vi "DeltaFour.vi"() -> ()   [LabVIEW 2012]
uses:
  <vilib>/NXT/Subs/MotorOutput.ctl
  <vilib>/NXT/NXT Controls/ConnectionType.ctl
  <vilib>/NXT/Block Support/NXT_InputPort.ctl
panel:
  in  "?":bool
  out "?":bool
  out "?":bool
  out "?":bool
  out "?":bool
  out "?":bool
  out "?":bool
  out "?":bool
  out "?":bool
  out "?":bool
  out "?":bool
  out "?":bool
  out "?":bool
  out "?":bool
  out "?":bool
  out "?":bool
  out "?":bool
  out "?":bool
  out "?":bool
  out "?":bool
  out "2D-Image":picture
  out "3D-Image":picture
  out "?":bool
  out "?":bool
  out "?":bool
  out "?":bool
  out "?":bool
  out "Progress":u8(slide) scale=0.0..100.0
  out "Motor B2":dbl
  out "Motor B1":dbl
  out "Motor A2":dbl
  out "Motor A1":dbl
  out "?":bool
  out "?":bool
  out "?":bool
  in  "Input molecule name or extended sum formula:":string
  out "Status:":string
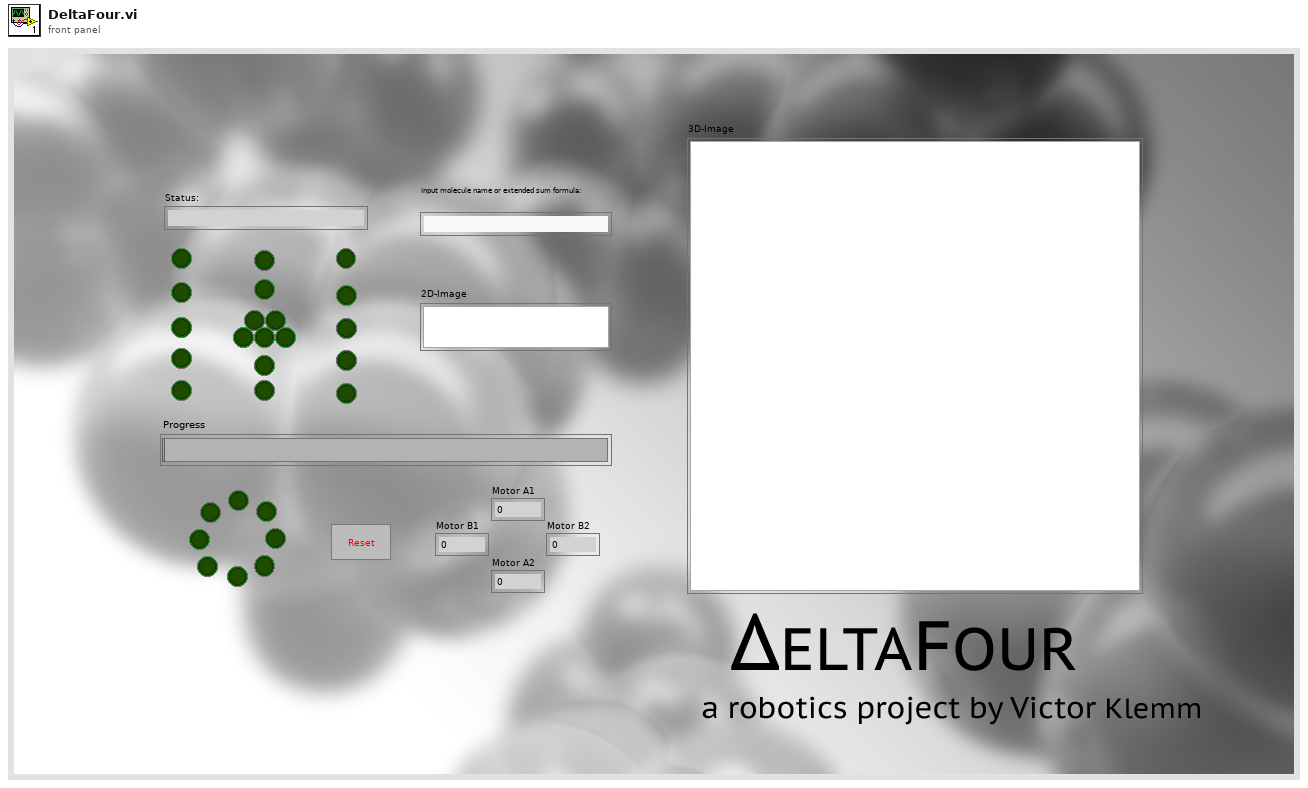
[diagram p1: front panel]
types:
  T1 = typedef "ConnectionType.ctl" = enum16{"Bluetooth", "USB", "WiFi"}
  T2 = typedef "LVHSConnector.ctl" = refnum<class "BrickReference.lvclass">
  T3 = typedef "imagedata.ctl" = cluster{"image type":i32, "image depth":i32, "image":u8[], "mask":u8[], "colors":u32[], "Rectangle":cluster{"left":i16, "top":i16, "right":i16, "bottom":i16}}
  T4 = typedef "MotorOutput.ctl" = u8
  T5 = typedef "NXT_InputPort.ctl" = u8
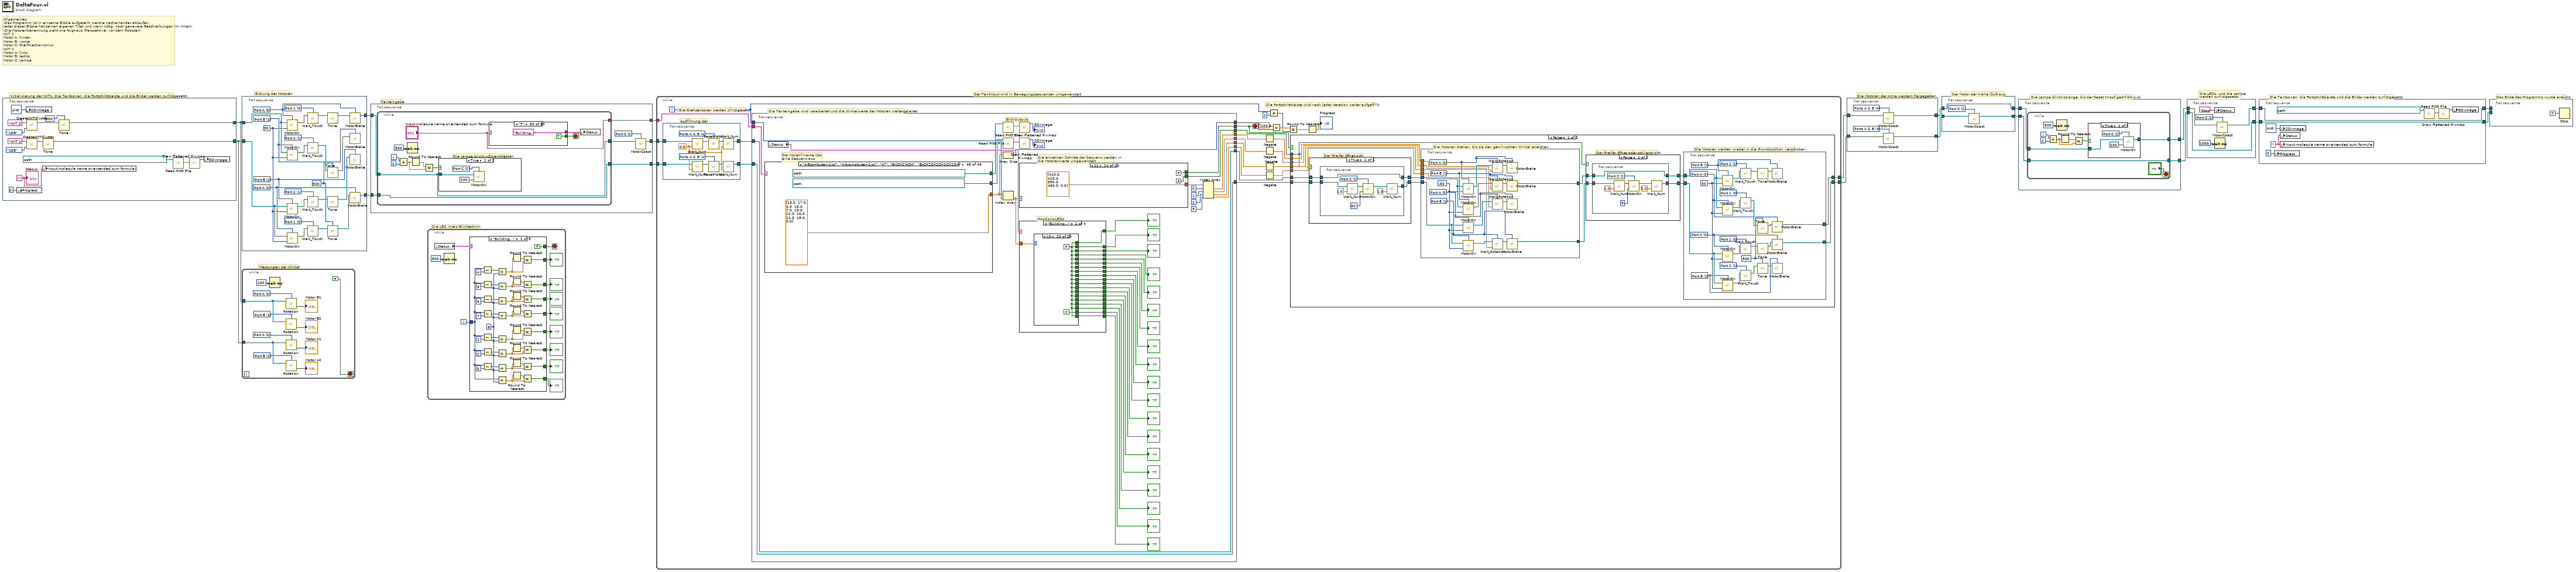
[diagram p0: block diagram]
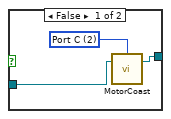
[diagram p2: hidden frame]
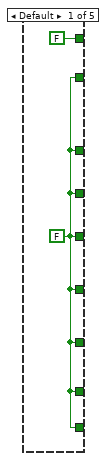
[diagram p3: hidden frame]
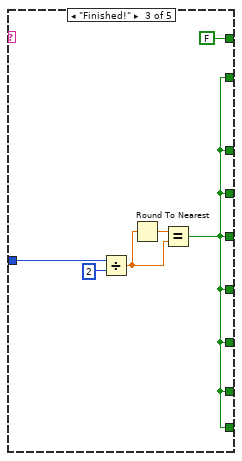
[diagram p4: hidden frame]
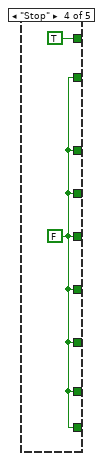
[diagram p5: hidden frame]
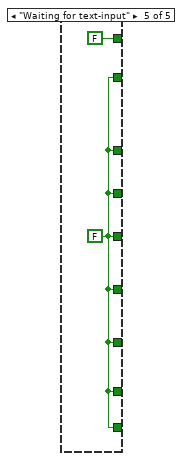
[diagram p6: hidden frame]
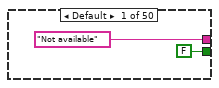
[diagram p7: hidden frame]
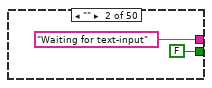
[diagram p8: hidden frame]
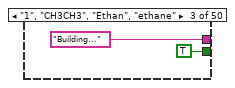
[diagram p9: hidden frame]
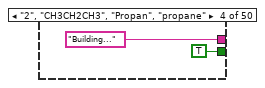
[diagram p10: hidden frame]
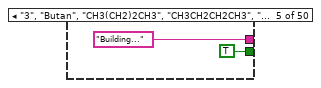
[diagram p11: hidden frame]
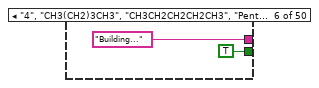
[diagram p12: hidden frame]
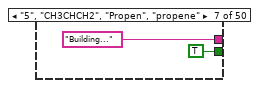
[diagram p13: hidden frame]
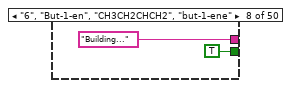
[diagram p14: hidden frame]
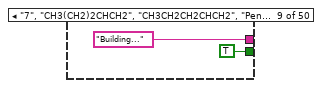
[diagram p15: hidden frame]
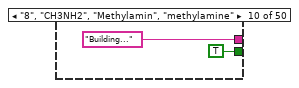
[diagram p16: hidden frame]
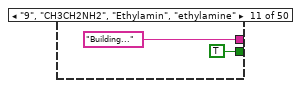
[diagram p17: hidden frame]
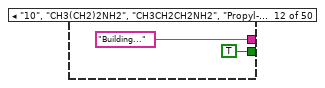
[diagram p18: hidden frame]
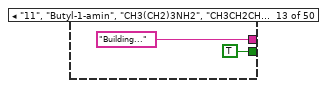
[diagram p19: hidden frame]
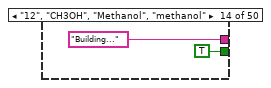
[diagram p20: hidden frame]
diagram:
  # "Eichung der Motoren"
  # "Der Textinput wird in Bewegungssequenzen umgewandelt"
  # "Die Textboxen, die Fortschrittsleiste und die Bilder werden zurŸckgesetzt."
  # "Das Ende des Programms wurde erreicht."
  # "Allgemeines:\n-Das Programm ist in einzelne Blšcke aufgeteilt, welche nacheinander ablaufen.\nJeder dieser Blšcke hat seinen eigenen Titel und wenn nštig, noch genauere Beschreibungen im Innern,\n-Die Motorenbenennung sieht wie folgt aus (Perspektive: vor dem Roboter):\nNXT 1\nMotor A: hinten\nMotor B: vorne\nMotor C: Greifmechanismus\nNXT 2\nMotor A: links\nMotor B: rechts\nMotor C: Lampe"
  # "Die Motoren der Arme werdem freigegeben."
  # "Die Lampe blinkt solange, bis der Reset Knopf gedrŸckt wird."
  # "Der Motor der Kralle lŠuft aus."
  # "Messungen der Winkel"
  # "Die LEDs, und die Lampe\nwerden zurŸckgesetzt"
  # "Texteingabe"
  # "Initialisierung der NXTs. Die Textboxen, die Fortschrittsleiste und die Bilder werden zurŸckgesetzt."
  # "Die LED -Kreis Blinktechnik"
  n1 = flat-sequence {
    tunnel: [w31] -> w10
    tunnel: [w29] -> w11
    frame #0 {
      w28 = "" ("Status:")
      n2 = local write "Progress"(u8 0 ("Progress")) -> ()
      n3 = local write "2D-Image"(picture data[5B] ("2D")) -> ()
      n4 = call <vilib>:"CreateNXTCluster.vi"("Connection Type"=ConnectionType."USB", "NXT name"="NXT 2") -> ("NXT"=w30:T2)  [unwired: 2 in]
      n5 = call <vilib>:"CreateNXTCluster.vi"("Connection Type"=ConnectionType."USB", "NXT name"="NXT 1") -> ("NXT"=w32:T2)  [unwired: 2 in]
      n6 = local write "Input molecule name or extended sum formula:"(w28) -> ()
      n7 = call <vilib>:"Tone.vi"("NXT"=w32) -> ("NXT"=w31:T2)  [unwired: 3 in]
      n8 = call <vilib>:"Tone.vi"("NXT"=w30, "Tone (440 Hz)"=u16 500) -> ("NXT"=w29:T2)  [unwired: 2 in]
      n9 = call <vilib>:"Read PNG File.vi"("path to PNG file"=path "/Macintosh HD/Users/victor_klemm/Documents/ÆFour Molecules/3D Molecules/0.png") -> ("image data"=w22:T3)  [unwired: 8 in, 2 out]
      n10 = call <vilib>:"Draw Flattened Pixmap.vi"("image data"=w22) -> ("new picture"=w20:picture)  [unwired: 8 in]
      n11 = local write "3D-Image"(w20) -> ()
      "Status:" <- w28
    }
  }
  n12 = flat-sequence {
    tunnel: w11 -> [w56]
    tunnel: w10 -> [w55]
    tunnel: [w42] -> w13
    tunnel: [w41] -> w12
    frame #0 {
      w35 = u16 500 ("Tone (440 Hz)")
      w38 = T4 1 items=["Port A"=0, "Port B"=1, "Port C"=2, "Ports A & B"=4, "Ports A & C"=5, "Ports B & C"=6, "All Ports"=3] ("Output Port (All Ports)")
      w51 = T5 1 items=["Port 1", "Port 2", "Port 3", "Port 4"] ("Port (Port 1)")
      w50 = T5 0 items=["Port 1", "Port 2", "Port 3", "Port 4"] ("Port (Port 1)")
      w36 = T4 1 items=["Port A"=0, "Port B"=1, "Port C"=2, "Ports A & B"=4, "Ports A & C"=5, "Ports B & C"=6, "All Ports"=3] ("Output Port (All Ports)")
      w37 = T4 0 items=["Port A"=0, "Port B"=1, "Port C"=2, "Ports A & B"=4, "Ports A & C"=5, "Ports B & C"=6, "All Ports"=3] ("Output Port (All Ports)")
      w39 = T5 1 items=["Port 1", "Port 2", "Port 3", "Port 4"] ("Port (Port 1)")
      w52 = T5 0 items=["Port 1", "Port 2", "Port 3", "Port 4"] ("Port (Port 1)")
      w43 = 30 ("Power (75)")
      w40 = T4 0 items=["Port A"=0, "Port B"=1, "Port C"=2, "Ports A & B"=4, "Ports A & C"=5, "Ports B & C"=6, "All Ports"=3] ("Output Port (All Ports)")
      n13 = call <vilib>:"MotorOn.vi"("Power (75)"=w43, "NXT"=w56, "Output Port (All Ports)"=w40) -> ("NXT"=w60:T2)  [unwired: 1 in]
      n14 = call <vilib>:"MotorOn.vi"("Power (75)"=w43, "NXT"=w56, "Output Port (All Ports)"=w38) -> ("NXT"=w59:T2)  [unwired: 1 in]
      n15 = call <vilib>:"MotorOn.vi"("Power (75)"=w43, "NXT"=w55, "Output Port (All Ports)"=w36) -> ("NXT"=w57:T2)  [unwired: 1 in]
      n16 = call <vilib>:"MotorOn.vi"("Power (75)"=w43, "NXT"=w55, "Output Port (All Ports)"=w37) -> ("NXT"=w58:T2)  [unwired: 1 in]
      n17 = call <vilib>:"Wait_Touch.vi"("NXT"=w60, "Port (Port 1)"=w52) -> ("NXT"=w54:T2)  [unwired: 2 in]
      n18 = call <vilib>:"Wait_Touch.vi"("NXT"=w59, "Port (Port 1)"=w39) -> ("NXT"=w49:T2)  [unwired: 2 in]
      n19 = call <vilib>:"Wait_Touch.vi"("NXT"=w57, "Port (Port 1)"=w51) -> ("NXT"=w47:T2)  [unwired: 2 in]
      n20 = call <vilib>:"Wait_Touch.vi"("NXT"=w58, "Port (Port 1)"=w50) -> ("NXT"=w45:T2)  [unwired: 2 in]
      n21 = call <vilib>:"Tone.vi"("NXT"=w54) -> ("NXT"=w53:T2)  [unwired: 3 in]
      n22 = call <vilib>:"Tone.vi"("NXT"=w49, "Tone (440 Hz)"=w35) -> ("NXT"=w48:T2)  [unwired: 2 in]
      n23 = call <vilib>:"Tone.vi"("NXT"=w47) -> ("NXT"=w46:T2)  [unwired: 3 in]
      n24 = call <vilib>:"Tone.vi"("NXT"=w45, "Tone (440 Hz)"=w35) -> ("NXT"=w44:T2)  [unwired: 2 in]
      n25 = call <vilib>:"MotorBrake.vi"("NXT"=w53, "Port (All Ports)"=w40) -> ("NXT"=w42:T2)  [unwired: 2 in]
      n26 = call <vilib>:"MotorBrake.vi"("NXT"=w48, "Port (All Ports)"=w38) -> ()  [unwired: 2 in, 1 out]
      n27 = call <vilib>:"MotorBrake.vi"("NXT"=w46, "Port (All Ports)"=w36) -> ()  [unwired: 2 in, 1 out]
      n28 = call <vilib>:"MotorBrake.vi"("NXT"=w44, "Port (All Ports)"=w37) -> ("NXT"=w41:T2)  [unwired: 2 in]
    }
  }
  n29 = while {
    tunnel: w11 -> [w68]
    tunnel: w10 -> [w67]
    stop <- FALSE stop-if-true
    w70 = T4 1 items=["Port A"=0, "Port B"=1, "Port C"=2, "Ports A & B"=4, "Ports A & C"=5, "Ports B & C"=6, "All Ports"=3] ("Output Port (All Ports)")
    w69 = T4 0 items=["Port A"=0, "Port B"=1, "Port C"=2, "Ports A & B"=4, "Ports A & C"=5, "Ports B & C"=6, "All Ports"=3] ("Output Port (All Ports)")
    w72 = T4 1 items=["Port A"=0, "Port B"=1, "Port C"=2, "Ports A & B"=4, "Ports A & C"=5, "Ports B & C"=6, "All Ports"=3] ("Output Port (All Ports)")
    w71 = T4 0 items=["Port A"=0, "Port B"=1, "Port C"=2, "Ports A & B"=4, "Ports A & C"=5, "Ports B & C"=6, "All Ports"=3] ("Output Port (All Ports)")
    n30 = Wait (ms)(milliseconds to wait=u32 100) -> ()  [unwired: 1 out]
    n31 = call <vilib>:"Rotation.vi"("NXT"=w68, "Port (Port A)"=w71) -> ("Angle of Rotation"=→"Motor B1":i32)  [unwired: 1 in, 1 out]
    n32 = call <vilib>:"Rotation.vi"("NXT"=w68, "Port (Port A)"=w72) -> ("Angle of Rotation"=→"Motor B2":i32)  [unwired: 1 in, 1 out]
    n33 = call <vilib>:"Rotation.vi"("NXT"=w67, "Port (Port A)"=w69) -> ("Angle of Rotation"=→"Motor A1":i32)  [unwired: 1 in, 1 out]
    n34 = call <vilib>:"Rotation.vi"("NXT"=w67, "Port (Port A)"=w70) -> ("Angle of Rotation"=→"Motor A2":i32)  [unwired: 1 in, 1 out]
  }
  n35 = flat-sequence {
    tunnel: w12 -> [w77]
    tunnel: [w79] -> w19
    tunnel: [w78] -> w8
    tunnel: [w74] -> w7
    tunnel: w13 -> [w76]
    frame #0 {
      w73 = T4 2 items=["Port A"=0, "Port B"=1, "Port C"=2, "Ports A & B"=4, "Ports A & C"=5, "Ports B & C"=6, "All Ports"=3] ("Port (All Ports)")
      n36 = while {
        tunnel: ["Input molecule name or extended sum formula:"] -> w79
        tunnel: [w89] -> w78
        tunnel: w77 -> [w89]
        tunnel: w76 -> [w84]
        tunnel: [w84] -> w75
        i -> [w83]
        stop <- w82 stop-if-true
        # "Die Lampe blinkt wŠhrenddessen"
        n37 = Divide(x=w83, y=2) -> (x/y=w86:dbl)
        n38 = Wait (ms)(milliseconds to wait=u32 500) -> ()  [unwired: 1 out]
        n39 = Round To Nearest(number=w86) -> (nearest integer value=w87:dbl)
        n40 = Equal?(x=w87, y=w86) -> (x = y?=w85:bool)
        n41 = case shown="True" w85 {
          tunnel: w84 -> [w191 w194]
          frame False {
            w192 = T4 2 items=["Port A"=0, "Port B"=1, "Port C"=2, "Ports A & B"=4, "Ports A & C"=5, "Ports B & C"=6, "All Ports"=3] ("Port (All Ports)")
            n42 = call <vilib>:"MotorCoast.vi"("NXT"=w191, "Port (All Ports)"=w192) -> ()  [unwired: 2 in, 1 out]
          }
          frame True {
            w193 = T4 2 items=["Port A"=0, "Port B"=1, "Port C"=2, "Ports A & B"=4, "Ports A & C"=5, "Ports B & C"=6, "All Ports"=3] ("Output Port (All Ports)")
            n43 = call <vilib>:"MotorOn.vi"("Power (75)"=100, "NXT"=w194, "Output Port (All Ports)"=w193) -> ()  [unwired: 1 in, 1 out]
          }
        }
        n44 = case shown="\"T\"" "Input molecule name or extended sum formula:" {
          tunnel: ["Not available" ("Status") "Waiting for text-input" ("Status") "Building..." ("Status") "Building..." ("Status") "Building..." ("Status") "Building..." ("Status") "Building..." ("Status") "Building..." ("Status") "Building..." ("Status") "Building..." ("Status") "Building..." ("Status") "Building..." ("Status") "Building..." ("Status") "Building..." ("Status") "Building..." ("Status") "Building..." ("Status") "Building..." ("Status") "Building..." ("Status") "Building..." ("Status") "Building..." ("Status") "Building..." ("Status") "Building..." ("Status") "Building..." ("Status") "Building..." ("Status") "Building..." ("Status") "Building..." ("Status") "Building..." ("Status") "Building..." ("Status") "Building..." ("Status") "Building..." ("Status") "Building..." ("Status") "Building..." ("Status") "Building..." ("Status") "Building..." ("Status") "Building..." ("Status") "Building..." ("Status") "Building..." ("Status") "Building..." ("Status") "Building..." ("Status") "Building..." ("Status") "Building..." ("Status") "Building..." ("Status") "Building..." ("Status") "Building..." ("Status") "Building..." ("Status") "Building..." ("Status") "Building..." ("Status") "Building..." ("Status") "Building..." ("Status") "Building..." ("Status")] -> w80
          tunnel: [FALSE FALSE TRUE TRUE TRUE TRUE TRUE TRUE TRUE TRUE TRUE TRUE TRUE TRUE TRUE TRUE TRUE TRUE TRUE TRUE TRUE TRUE TRUE TRUE TRUE TRUE TRUE TRUE TRUE TRUE TRUE TRUE TRUE TRUE TRUE TRUE TRUE TRUE TRUE TRUE TRUE TRUE TRUE TRUE TRUE TRUE TRUE TRUE TRUE TRUE] -> w82
          frame Default {
          }
          frame "" {
          }
          frame "1", "CH3CH3", "Ethan", "ethane" {
          }
          frame "2", "CH3CH2CH3", "Propan", "propane" {
          }
          frame "3", "Butan", "CH3(CH2)2CH3", "CH3CH2CH2CH3", "butane" {
          }
          frame "4", "CH3(CH2)3CH3", "CH3CH2CH2CH2CH3", "Pentan", "pentane" {
          }
          frame "5", "CH3CHCH2", "Propen", "propene" {
          }
          frame "6", "But-1-en", "CH3CH2CHCH2", "but-1-ene" {
          }
          frame "7", "CH3(CH2)2CHCH2", "CH3CH2CH2CHCH2", "Pent-1-en", "pent-1-ene" {
          }
          frame "8", "CH3NH2", "Methylamin", "methylamine" {
          }
          frame "9", "CH3CH2NH2", "Ethylamin", "ethylamine" {
          }
          frame "10", "CH3(CH2)2NH2", "CH3CH2CH2NH2", "Propyl-1-amin", "propyl-1-amine" {
          }
          frame "11", "Butyl-1-amin", "CH3(CH2)3NH2", "CH3CH2CH2CH2NH2", "butyl-1-amine" {
          }
          frame "12", "CH3OH", "Methanol", "methanol" {
          }
          frame "13", "CH3CH2OH", "Ethanol", "ethanol" {
          }
          frame "14", "CH3(CH2)2OH", "CH3CH2CH2OH", "Propanol", "propanol" {
          }
          frame "15", "Butanol", "CH3(CH2)3OH", "CH3CH2CH2CH2OH", "butanol" {
          }
          frame "16", "CH3CH2Cl", "Chlorethan", "chloroethane" {
          }
          frame "1-Chlorpropan", "1-chloropropane", "17", "CH3(CH2)2Cl", "CH3CH2CH2Cl" {
          }
          frame "1-Chlorbutan", "1-chlorobutane", "18", "CH3(CH2)3Cl", "CH3CH2CH2CH2Cl" {
          }
          frame "1-Chlorpentan", "1-chloropentane", "19", "CH3(CH2)4Cl", "CH3CH2CH2CH2CH2Cl" {
          }
          frame "20", "CH3CH2I", "Iodethan", "iodoethane" {
          }
          frame "1-Iodpropan", "1-iodopropane", "21", "CH3(CH2)2I", "CH3CH2CH2I" {
          }
          frame "1-Iodbutan", "1-iodobutane", "22", "CH3(CH2)3I", "CH3CH2CH2CH2I" {
          }
          frame "1-Iodpentan", "1-iodopentane", "23", "CH3(CH2)4I", "CH3CH2CH2CH2CH2I" {
          }
          frame "24", "Bromethan", "CH3CH2Br", "bromoethane" {
          }
          frame "1-Brompropan", "1-bromopropane", "25", "CH3(CH2)2Br", "CH3CH2CH2Br" {
          }
          frame "1-Brombutan", "1-bromobutane", "26", "CH3(CH2)3Br", "CH3CH2CH2CH2Br" {
          }
          frame "1-Brompentan", "1-bromopentane", "27", "CH3(CH2)4Br", "CH3CH2CH2CH2CH2Br" {
          }
          frame "28", "CH2CHNH2", "Ethenylamin", "ethenylamine" {
          }
          frame "29", "But-3-enyl-1-amin", "CH2CH(CH2)2NH2", "CH2CHCH2CH2NH2", "but-3-enyl-1-amine" {
          }
          frame "30", "CH2CHOH", "Ethenol", "ethenol" {
          }
          frame "31", "But-3-en-1-ol", "CH2CH(CH2)2OH", "CH2CHCH2CH2OH", "but-3-en-1-ol" {
          }
          frame "3-Chlorprop-1-en", "3-chloroprop-1-ene", "32", "CH2CHCH2Cl" {
          }
          frame "33", "5-Chlorpent-1-en", "5-chloropent-1-ene", "CH2CH(CH2)3Cl", "CH2CHCH2CH2CH2Cl" {
          }
          frame "3-Iodprop-1-en", "3-iodoprop-1-ene", "34", "CH2CHCH2I" {
          }
          frame "35", "5-Iodpent-1-en", "5-iodopent-1-ene", "CH2CH(CH2)3I", "CH2CHCH2CH2CH2I" {
          }
          frame "3-Bromprop-1-en", "3-bromoprop-1-ene", "36", "CH2CHCH2Br" {
          }
          frame "37", "5-Brompent-1-en", "5-bromopent-1-ene", "CH2CH(CH2)3Br", "CH2CHCH2CH2CH2Br" {
          }
          frame "38", "Aminomethanol", "NH2CH2OH", "aminomethanol" {
          }
          frame "3-Aminopropan-1-ol", "3-aminopropan-1-ol", "39", "NH2(CH2)3OH", "NH2CH2CH2CH2OH" {
          }
          frame "40", "Methandiol", "OHCH2OH", "methanediol" {
          }
          frame "41", "OH(CH2)3OH", "OHCH2CH2CH2OH", "Propan-1,3-diol", "propane-1,3-diol" {
          }
          frame "2-Chlorethan-1-ol", "2-chloroethan-1-ol", "42", "ClCH2CH2OH" {
          }
          frame "4-Chlorbutan-1-ol", "4-chlorobutan-1-ol", "43", "Cl(CH2)4OH", "ClCH2CH2CH2CH2OH" {
          }
          frame "2-Iodethan-1-ol", "2-iodoethan-1-ol", "44", "ICH2CH2OH" {
          }
          frame "4-Iodbutan-1-ol", "4-iodobutan-1-ol", "45", "I(CH2)4OH", "ICH2CH2CH2CH2OH" {
          }
          frame "2-Bromethan-1-ol", "2-bromoethan-1-ol", "46", "BrCH2CH2OH" {
          }
          frame "4-Brombutan-1-ol", "4-bromobutan-1-ol", "47", "Br(CH2)4OH", "BrCH2CH2CH2CH2OH" {
          }
          frame "T" {
          }
        }
        n45 = local write "Status:"(w80) -> ()
      }
      n46 = call <vilib>:"MotorCoast.vi"("NXT"=w75, "Port (All Ports)"=w73) -> ("NXT"=w74:T2)  [unwired: 2 in]
    }
  }
  n47 = while {
    i -> [w207]
    stop <- w205 stop-if-true
    n48 = local read "Status:"() -> (w204:string)
    n49 = Wait (ms)(milliseconds to wait=u32 500) -> ()  [unwired: 1 out]
    n50 = case shown="\"Building...\"" w204 {
      tunnel: w207 -> [_ w211 w253 _ _]
      tunnel: [FALSE FALSE FALSE TRUE FALSE] -> w205
      tunnel: [w208 w239 w251 w257 w259] -> w203
      tunnel: [w208 w238 w251 w257 w259] -> w202
      tunnel: [w208 w237 w251 w257 w259] -> w201
      tunnel: [w208 w232 w251 w257 w259] -> w200
      tunnel: [w208 w228 w251 w257 w259] -> w199
      tunnel: [w208 w222 w251 w257 w259] -> w198
      tunnel: [w208 w217 w251 w257 w259] -> w197
      tunnel: [w208 w212 w251 w257 w259] -> w196
      frame Default {
        w208 = FALSE ("stop? (T)")
      }
      frame "Building..." {
        w210 = 8 ("y")
        n51 = Subtract(x=w211, y=4) -> (x-y=w230:i32)
        n52 = Subtract(x=w211, y=5) -> (x-y=w225:i32)
        n53 = Subtract(x=w211, y=6) -> (x-y=w220:i32)
        n54 = Subtract(x=w211, y=7) -> (x-y=w215:i32)
        n55 = Subtract(x=w211, y=1) -> (x-y=w246:i32)
        n56 = Subtract(x=w211, y=2) -> (x-y=w242:i32)
        n57 = Subtract(x=w211, y=3) -> (x-y=w234:i32)
        n58 = Divide(x=w230, y=w210) -> (x/y=w231:dbl)
        n59 = Divide(x=w225, y=w210) -> (x/y=w226:dbl)
        n60 = Divide(x=w220, y=w210) -> (x/y=w221:dbl)
        n61 = Divide(x=w215, y=w210) -> (x/y=w216:dbl)
        n62 = Divide(x=w246, y=w210) -> (x/y=w247:dbl)
        n63 = Divide(x=w242, y=w210) -> (x/y=w243:dbl)
        n64 = Divide(x=w234, y=w210) -> (x/y=w235:dbl)
        n65 = Divide(x=w211, y=w210) -> (x/y=w249:dbl)
        n66 = Round To Nearest(number=w231) -> (nearest integer value=w227:dbl)
        n67 = Round To Nearest(number=w226) -> (nearest integer value=w223:dbl)
        n68 = Round To Nearest(number=w221) -> (nearest integer value=w218:dbl)
        n69 = Round To Nearest(number=w216) -> (nearest integer value=w213:dbl)
        n70 = Round To Nearest(number=w247) -> (nearest integer value=w248:dbl)
        n71 = Round To Nearest(number=w243) -> (nearest integer value=w244:dbl)
        n72 = Round To Nearest(number=w235) -> (nearest integer value=w236:dbl)
        n73 = Round To Nearest(number=w249) -> (nearest integer value=w250:dbl)
        n74 = Equal?(x=w227, y=w231) -> (x = y?=w228:bool)
        n75 = Equal?(x=w223, y=w226) -> (x = y?=w222:bool)
        n76 = Equal?(x=w218, y=w221) -> (x = y?=w217:bool)
        n77 = Equal?(x=w213, y=w216) -> (x = y?=w212:bool)
        n78 = Equal?(x=w248, y=w247) -> (x = y?=w237:bool)
        n79 = Equal?(x=w244, y=w243) -> (x = y?=w238:bool)
        n80 = Equal?(x=w236, y=w235) -> (x = y?=w232:bool)
        n81 = Equal?(x=w250, y=w249) -> (x = y?=w239:bool)
      }
      frame "Finished!" {
        n82 = Divide(x=w253, y=2) -> (x/y=w255:dbl)
        n83 = Round To Nearest(number=w255) -> (nearest integer value=w252:dbl)
        n84 = Equal?(x=w252, y=w255) -> (x = y?=w251:bool)
      }
      frame "Stop" {
        w257 = FALSE ("stop? (T)")
      }
      frame "Waiting for text-input" {
        w259 = FALSE ("stop? (T)")
      }
    }
    "?" <- w203
    "?" <- w202
    "?" <- w201
    "?" <- w197
    "?" <- w196
    "?" <- w200
    "?" <- w199
    "?" <- w198
  }
  n85 = while {
    tunnel: w8 -> [w285]
    tunnel: w7 -> [w284]
    tunnel: w19 -> [w281]
    tunnel: [w262] -> w4
    tunnel: [w261] -> w5
    i -> [w273]
    stop <- w279 stop-if-true
    # "Die Fortschrittsleiste wird nach jeder Iteration weiter aufgefŸllt."
    # "AusfŸhrung der"
    # "Die Texteingabe wird verarbeitet und die Winkelwerte der Motoren weitergeleitet"
    # "Die Drehsensoren werden zŸrickgesetzt"
    n86 = flat-sequence {
      tunnel: w285 -> [w726]
      tunnel: [w721] -> w283
      tunnel: [w720] -> w282
      tunnel: w284 -> [w719]
      frame #0 {
        w722 = sgl 0.5 ("Time (1 sec)")
        w728 = T4 4 items=["Port A"=0, "Port B"=1, "Port C"=2, "Ports A & B"=4, "Ports A & C"=5, "Ports B & C"=6, "All Ports"=3] ("Port (All Ports)")
        w729 = T4 4 items=["Port A"=0, "Port B"=1, "Port C"=2, "Ports A & B"=4, "Ports A & C"=5, "Ports B & C"=6, "All Ports"=3] ("Port (All Ports)")
        n87 = call <vilib>:"Wait_Num.vi"("Time (1 sec)"=w722, "NXT"=w719) -> ("NXT"=w727:T2)  [unwired: 2 in]
        n88 = call <vilib>:"Wait_Num.vi"("Time (1 sec)"=w722, "NXT"=w726) -> ("NXT"=w725:T2)  [unwired: 2 in]
        n89 = call <vilib>:"ResetMotor.vi"("NXT"=w727, "Port (All Ports)"=w728) -> ("NXT"=w723:T2)  [unwired: 2 in]
        n90 = call <vilib>:"ResetMotor.vi"("NXT"=w725, "Port (All Ports)"=w729) -> ("NXT"=w724:T2)  [unwired: 2 in]
        n91 = call <vilib>:"Wait_Num.vi"("Time (1 sec)"=w722, "NXT"=w723) -> ("NXT"=w720:T2)  [unwired: 2 in]
        n92 = call <vilib>:"Wait_Num.vi"("Time (1 sec)"=w722, "NXT"=w724) -> ("NXT"=w721:T2)  [unwired: 2 in]
      }
    }
    n93 = flat-sequence {
      tunnel: [w432] -> w264
      tunnel: [w431] -> w270
      tunnel: [w430] -> w268
      tunnel: [w429] -> w266
      tunnel: [w425] -> w287
      tunnel: w283 -> [w425]
      tunnel: w282 -> [w428]
      tunnel: [w428] -> w286
      tunnel: w281 -> [w427]
      tunnel: w273 -> [w423]
      tunnel: [w426] -> w279
      tunnel: [w424] -> w280
      tunnel: [w422] -> w274
      frame #0 {
        # "Positions-LEDs"
        # "Bild-Outputs"
        # "Die einzelnen Schritte der Sequenz werden in\ndie Motorenwerte umgewandelt"
        # "Der MolekŸlname lšst eine Sequenz aus"
        n94 = case shown="\"4-Brombutan-1-ol\", \"4-bromobutan-1-ol\", \"47\", \"Br(CH2)4OH\", \"BrCH2CH2CH2CH2OH\"" w427 {
          tunnel: [dbl[] [0.0] ("array") dbl[] [1.0, 15.0, 6.0, 16.0, 0.0] ("array") dbl[] [10.0, 17.0, 1.0, 15.0, 12.0, 16.0, 0.0] ("array") dbl[] [13.0, 17.0, 1.0, 15.0, 12.0, 16.0, 6.0, 18.0, 0.0] ("array") dbl[] [13.0, 17.0, 1.0, 15.0, 10.0, 19.0, 12.0, 16.0, 11.0, 18.0, 0.0] ("array") dbl[] [10.0, 17.0, 9.0, 15.0, 8.0, 16.0, 0.0] ("array") dbl[] [13.0, 17.0, 9.0, 15.0, 8.0, 16.0, 6.0, 18.0, 0.0] ("array") dbl[] [13.0, 17.0, 9.0, 15.0, 10.0, 19.0, 8.0, 16.0, 12.0, 18.0, 0.0] ("array") dbl[] [5.0, 15.0, 6.0, 16.0, 0.0] ("array") dbl[] [10.0, 17.0, 5.0, 15.0, 12.0, 16.0, 0.0] ("array") dbl[] [13.0, 17.0, 5.0, 15.0, 12.0, 16.0, 6.0, 18.0, 0.0] ("array") dbl[] [13.0, 17.0, 5.0, 15.0, 10.0, 19.0, 12.0, 16.0, 11.0, 18.0, 0.0] ("array") dbl[] [14.0, 20.0, 6.0, 16.0, 0.0] ("array") dbl[] [10.0, 17.0, 14.0, 20.0, 12.0, 16.0, 0.0] ("array") dbl[] [13.0, 17.0, 14.0, 20.0, 12.0, 16.0, 6.0, 18.0, 0.0] ("array") dbl[] [13.0, 17.0, 14.0, 15.0, 10.0, 19.0, 12.0, 16.0, 11.0, 18.0, 0.0] ("array") dbl[] [2.0, 15.0, 6.0, 16.0, 0.0] ("array") dbl[] [10.0, 17.0, 2.0, 15.0, 12.0, 16.0, 0.0] ("array") dbl[] [13.0, 17.0, 2.0, 15.0, 12.0, 16.0, 6.0, 18.0, 0.0] ("array") dbl[] [13.0, 17.0, 2.0, 15.0, 10.0, 19.0, 12.0, 16.0, 11.0, 18.0, 0.0] ("array") dbl[] [3.0, 15.0, 6.0, 16.0, 0.0] ("array") dbl[] [10.0, 17.0, 3.0, 15.0, 12.0, 16.0, 0.0] ("array") dbl[] [13.0, 17.0, 3.0, 15.0, 12.0, 16.0, 6.0, 18.0, 0.0] ("array") dbl[] [13.0, 17.0, 3.0, 15.0, 10.0, 19.0, 12.0, 16.0, 11.0, 18.0, 0.0] ("array") dbl[] [4.0, 15.0, 6.0, 16.0, 0.0] ("array") dbl[] [10.0, 17.0, 4.0, 15.0, 12.0, 16.0, 0.0] ("array") dbl[] [13.0, 17.0, 4.0, 15.0, 12.0, 16.0, 6.0, 18.0, 0.0] ("array") dbl[] [13.0, 17.0, 4.0, 15.0, 10.0, 19.0, 12.0, 16.0, 11.0, 18.0, 0.0] ("array") dbl[] [9.0, 19.0, 5.0, 17.0, 8.0, 18.0, 0.0] ("array") dbl[] [13.0, 17.0, 5.0, 15.0, 9.0, 19.0, 12.0, 16.0, 8.0, 18.0, 0.0] ("array") dbl[] [14.0, 17.0, 9.0, 19.0, 8.0, 21.0, 0.0] ("array") dbl[] [13.0, 17.0, 14.0, 20.0, 9.0, 19.0, 12.0, 22.0, 8.0, 21.0] ("array") dbl[] [2.0, 17.0, 9.0, 19.0, 8.0, 18.0, 0.0] ("array") dbl[] [13.0, 17.0, 2.0, 15.0, 9.0, 19.0, 12.0, 16.0, 8.0, 18.0, 0.0] ("array") dbl[] [3.0, 17.0, 9.0, 19.0, 8.0, 18.0, 0.0] ("array") dbl[] [13.0, 17.0, 3.0, 15.0, 9.0, 19.0, 12.0, 16.0, 8.0, 18.0, 0.0] ("array") dbl[] [4.0, 17.0, 9.0, 19.0, 8.0, 18.0, 0.0] ("array") dbl[] [13.0, 17.0, 4.0, 15.0, 9.0, 19.0, 12.0, 16.0, 8.0, 18.0, 0.0] ("array") dbl[] [5.0, 17.0, 7.0, 19.0, 12.0, 18.0, 0.0] ("array") dbl[] [13.0, 17.0, 5.0, 15.0, 7.0, 19.0, 12.0, 16.0, 11.0, 18.0, 0.0] ("array") dbl[] [7.0, 17.0, 14.0, 20.0, 12.0, 16.0, 0.0] ("array") dbl[] [13.0, 17.0, 14.0, 20.0, 7.0, 19.0, 12.0, 16.0, 11.0, 18.0, 0.0] ("array") dbl[] [2.0, 17.0, 7.0, 19.0, 12.0, 18.0, 0.0] ("array") dbl[] [13.0, 17.0, 2.0, 15.0, 7.0, 19.0, 12.0, 16.0, 11.0, 18.0, 0.0] ("array") dbl[] [3.0, 17.0, 7.0, 19.0, 12.0, 18.0, 0.0] ("array") dbl[] [13.0, 17.0, 3.0, 15.0, 7.0, 19.0, 12.0, 16.0, 11.0, 18.0, 0.0] ("array") dbl[] [4.0, 17.0, 7.0, 19.0, 12.0, 18.0, 0.0] ("array") dbl[] [13.0, 17.0, 4.0, 15.0, 7.0, 19.0, 12.0, 16.0, 11.0, 18.0, 0.0] ("array") dbl[] [9.0, 23.0, 0.0, 0.0, 0.0] ("array")] -> w420
          tunnel: [path "" ("path to PNG file") path "/Macintosh HD/Users/victor_klemm/Documents/ÆFour Molecules/2D Molecules/1.png" ("path to PNG file") path "/Macintosh HD/Users/victor_klemm/Documents/ÆFour Molecules/2D Molecules/2.png" ("path to PNG file") path "/Macintosh HD/Users/victor_klemm/Documents/ÆFour Molecules/2D Molecules/3.png" ("path to PNG file") path "/Macintosh HD/Users/victor_klemm/Documents/ÆFour Molecules/2D Molecules/4.png" ("path to PNG file") path "/Macintosh HD/Users/victor_klemm/Documents/ÆFour Molecules/2D Molecules/5.png" ("path to PNG file") path "/Macintosh HD/Users/victor_klemm/Documents/ÆFour Molecules/2D Molecules/6.png" ("path to PNG file") path "/Macintosh HD/Users/victor_klemm/Documents/ÆFour Molecules/2D Molecules/7.png" ("path to PNG file") path "/Macintosh HD/Users/victor_klemm/Documents/ÆFour Molecules/2D Molecules/8.png" ("path to PNG file") path "/Macintosh HD/Users/victor_klemm/Documents/ÆFour Molecules/2D Molecules/9.png" ("path to PNG file") path "/Macintosh HD/Users/victor_klemm/Documents/ÆFour Molecules/2D Molecules/10.png" ("path to PNG file") path "/Macintosh HD/Users/victor_klemm/Documents/ÆFour Molecules/2D Molecules/11.png" ("path to PNG file") path "/Macintosh HD/Users/victor_klemm/Documents/ÆFour Molecules/2D Molecules/12.png" ("path to PNG file") path "/Macintosh HD/Users/victor_klemm/Documents/ÆFour Molecules/2D Molecules/13.png" ("path to PNG file") path "/Macintosh HD/Users/victor_klemm/Documents/ÆFour Molecules/2D Molecules/14.png" ("path to PNG file") path "/Macintosh HD/Users/victor_klemm/Documents/ÆFour Molecules/2D Molecules/15.png" ("path to PNG file") path "/Macintosh HD/Users/victor_klemm/Documents/ÆFour Molecules/2D Molecules/16.png" ("path to PNG file") path "/Macintosh HD/Users/victor_klemm/Documents/ÆFour Molecules/2D Molecules/17.png" ("path to PNG file") path "/Macintosh HD/Users/victor_klemm/Documents/ÆFour Molecules/2D Molecules/18.png" ("path to PNG file") path "/Macintosh HD/Users/victor_klemm/Documents/ÆFour Molecules/2D Molecules/19.png" ("path to PNG file") path "/Macintosh HD/Users/victor_klemm/Documents/ÆFour Molecules/2D Molecules/20.png" ("path to PNG file") path "/Macintosh HD/Users/victor_klemm/Documents/ÆFour Molecules/2D Molecules/21.png" ("path to PNG file") path "/Macintosh HD/Users/victor_klemm/Documents/ÆFour Molecules/2D Molecules/22.png" ("path to PNG file") path "/Macintosh HD/Users/victor_klemm/Documents/ÆFour Molecules/2D Molecules/23.png" ("path to PNG file") path "/Macintosh HD/Users/victor_klemm/Documents/ÆFour Molecules/2D Molecules/24.png" ("path to PNG file") path "/Macintosh HD/Users/victor_klemm/Documents/ÆFour Molecules/2D Molecules/25.png" ("path to PNG file") path "/Macintosh HD/Users/victor_klemm/Documents/ÆFour Molecules/2D Molecules/26.png" ("path to PNG file") path "/Macintosh HD/Users/victor_klemm/Documents/ÆFour Molecules/2D Molecules/27.png" ("path to PNG file") path "/Macintosh HD/Users/victor_klemm/Documents/ÆFour Molecules/2D Molecules/28.png" ("path to PNG file") path "/Macintosh HD/Users/victor_klemm/Documents/ÆFour Molecules/2D Molecules/29.png" ("path to PNG file") path "/Macintosh HD/Users/victor_klemm/Documents/ÆFour Molecules/2D Molecules/30.png" ("path to PNG file") path "/Macintosh HD/Users/victor_klemm/Documents/ÆFour Molecules/2D Molecules/31.png" ("path to PNG file") path "/Macintosh HD/Users/victor_klemm/Documents/ÆFour Molecules/2D Molecules/32.png" ("path to PNG file") path "/Macintosh HD/Users/victor_klemm/Documents/ÆFour Molecules/2D Molecules/33.png" ("path to PNG file") path "/Macintosh HD/Users/victor_klemm/Documents/ÆFour Molecules/2D Molecules/34.png" ("path to PNG file") path "/Macintosh HD/Users/victor_klemm/Documents/ÆFour Molecules/2D Molecules/35.png" ("path to PNG file") path "/Macintosh HD/Users/victor_klemm/Documents/ÆFour Molecules/2D Molecules/36.png" ("path to PNG file") path "/Macintosh HD/Users/victor_klemm/Documents/ÆFour Molecules/2D Molecules/37.png" ("path to PNG file") path "/Macintosh HD/Users/victor_klemm/Documents/ÆFour Molecules/2D Molecules/38.png" ("path to PNG file") path "/Macintosh HD/Users/victor_klemm/Documents/ÆFour Molecules/2D Molecules/39.png" ("path to PNG file") path "/Macintosh HD/Users/victor_klemm/Documents/ÆFour Molecules/2D Molecules/40.png" ("path to PNG file") path "/Macintosh HD/Users/victor_klemm/Documents/ÆFour Molecules/2D Molecules/41.png" ("path to PNG file") path "/Macintosh HD/Users/victor_klemm/Documents/ÆFour Molecules/2D Molecules/42.png" ("path to PNG file") path "/Macintosh HD/Users/victor_klemm/Documents/ÆFour Molecules/2D Molecules/43.png" ("path to PNG file") path "/Macintosh HD/Users/victor_klemm/Documents/ÆFour Molecules/2D Molecules/44.png" ("path to PNG file") path "/Macintosh HD/Users/victor_klemm/Documents/ÆFour Molecules/2D Molecules/45.png" ("path to PNG file") path "/Macintosh HD/Users/victor_klemm/Documents/ÆFour Molecules/2D Molecules/46.png" ("path to PNG file") path "/Macintosh HD/Users/victor_klemm/Documents/ÆFour Molecules/2D Molecules/47.png" ("path to PNG file") path "/Macintosh HD/Users/victor_klemm/Documents/ÆFour Molecules/2D Molecules/16.png" ("path to PNG file")] -> w415
          tunnel: [path "" ("path to PNG file") path "/Macintosh HD/Users/victor_klemm/Documents/ÆFour Molecules/3D Molecules/1.png" ("path to PNG file") path "/Macintosh HD/Users/victor_klemm/Documents/ÆFour Molecules/3D Molecules/2.png" ("path to PNG file") path "/Macintosh HD/Users/victor_klemm/Documents/ÆFour Molecules/3D Molecules/3.png" ("path to PNG file") path "/Macintosh HD/Users/victor_klemm/Documents/ÆFour Molecules/3D Molecules/4.png" ("path to PNG file") path "/Macintosh HD/Users/victor_klemm/Documents/ÆFour Molecules/3D Molecules/5.png" ("path to PNG file") path "/Macintosh HD/Users/victor_klemm/Documents/ÆFour Molecules/3D Molecules/6.png" ("path to PNG file") path "/Macintosh HD/Users/victor_klemm/Documents/ÆFour Molecules/3D Molecules/7.png" ("path to PNG file") path "/Macintosh HD/Users/victor_klemm/Documents/ÆFour Molecules/3D Molecules/8.png" ("path to PNG file") path "/Macintosh HD/Users/victor_klemm/Documents/ÆFour Molecules/3D Molecules/9.png" ("path to PNG file") path "/Macintosh HD/Users/victor_klemm/Documents/ÆFour Molecules/3D Molecules/10.png" ("path to PNG file") path "/Macintosh HD/Users/victor_klemm/Documents/ÆFour Molecules/3D Molecules/11.png" ("path to PNG file") path "/Macintosh HD/Users/victor_klemm/Documents/ÆFour Molecules/3D Molecules/12.png" ("path to PNG file") path "/Macintosh HD/Users/victor_klemm/Documents/ÆFour Molecules/3D Molecules/13.png" ("path to PNG file") path "/Macintosh HD/Users/victor_klemm/Documents/ÆFour Molecules/3D Molecules/14.png" ("path to PNG file") path "/Macintosh HD/Users/victor_klemm/Documents/ÆFour Molecules/3D Molecules/15.png" ("path to PNG file") path "/Macintosh HD/Users/victor_klemm/Documents/ÆFour Molecules/3D Molecules/16.png" ("path to PNG file") path "/Macintosh HD/Users/victor_klemm/Documents/ÆFour Molecules/3D Molecules/17.png" ("path to PNG file") path "/Macintosh HD/Users/victor_klemm/Documents/ÆFour Molecules/3D Molecules/18.png" ("path to PNG file") path "/Macintosh HD/Users/victor_klemm/Documents/ÆFour Molecules/3D Molecules/19.png" ("path to PNG file") path "/Macintosh HD/Users/victor_klemm/Documents/ÆFour Molecules/3D Molecules/20.png" ("path to PNG file") path "/Macintosh HD/Users/victor_klemm/Documents/ÆFour Molecules/3D Molecules/21.png" ("path to PNG file") path "/Macintosh HD/Users/victor_klemm/Documents/ÆFour Molecules/3D Molecules/22.png" ("path to PNG file") path "/Macintosh HD/Users/victor_klemm/Documents/ÆFour Molecules/3D Molecules/23.png" ("path to PNG file") path "/Macintosh HD/Users/victor_klemm/Documents/ÆFour Molecules/3D Molecules/24.png" ("path to PNG file") path "/Macintosh HD/Users/victor_klemm/Documents/ÆFour Molecules/3D Molecules/25.png" ("path to PNG file") path "/Macintosh HD/Users/victor_klemm/Documents/ÆFour Molecules/3D Molecules/26.png" ("path to PNG file") path "/Macintosh HD/Users/victor_klemm/Documents/ÆFour Molecules/3D Molecules/27.png" ("path to PNG file") path "/Macintosh HD/Users/victor_klemm/Documents/ÆFour Molecules/3D Molecules/28.png" ("path to PNG file") path "/Macintosh HD/Users/victor_klemm/Documents/ÆFour Molecules/3D Molecules/29.png" ("path to PNG file") path "/Macintosh HD/Users/victor_klemm/Documents/ÆFour Molecules/3D Molecules/30.png" ("path to PNG file") path "/Macintosh HD/Users/victor_klemm/Documents/ÆFour Molecules/3D Molecules/31.png" ("path to PNG file") path "/Macintosh HD/Users/victor_klemm/Documents/ÆFour Molecules/3D Molecules/32.png" ("path to PNG file") path "/Macintosh HD/Users/victor_klemm/Documents/ÆFour Molecules/3D Molecules/33.png" ("path to PNG file") path "/Macintosh HD/Users/victor_klemm/Documents/ÆFour Molecules/3D Molecules/34.png" ("path to PNG file") path "/Macintosh HD/Users/victor_klemm/Documents/ÆFour Molecules/3D Molecules/35.png" ("path to PNG file") path "/Macintosh HD/Users/victor_klemm/Documents/ÆFour Molecules/3D Molecules/36.png" ("path to PNG file") path "/Macintosh HD/Users/victor_klemm/Documents/ÆFour Molecules/3D Molecules/37.png" ("path to PNG file") path "/Macintosh HD/Users/victor_klemm/Documents/ÆFour Molecules/3D Molecules/38.png" ("path to PNG file") path "/Macintosh HD/Users/victor_klemm/Documents/ÆFour Molecules/3D Molecules/39.png" ("path to PNG file") path "/Macintosh HD/Users/victor_klemm/Documents/ÆFour Molecules/3D Molecules/40.png" ("path to PNG file") path "/Macintosh HD/Users/victor_klemm/Documents/ÆFour Molecules/3D Molecules/41.png" ("path to PNG file") path "/Macintosh HD/Users/victor_klemm/Documents/ÆFour Molecules/3D Molecules/42.png" ("path to PNG file") path "/Macintosh HD/Users/victor_klemm/Documents/ÆFour Molecules/3D Molecules/43.png" ("path to PNG file") path "/Macintosh HD/Users/victor_klemm/Documents/ÆFour Molecules/3D Molecules/44.png" ("path to PNG file") path "/Macintosh HD/Users/victor_klemm/Documents/ÆFour Molecules/3D Molecules/45.png" ("path to PNG file") path "/Macintosh HD/Users/victor_klemm/Documents/ÆFour Molecules/3D Molecules/46.png" ("path to PNG file") path "/Macintosh HD/Users/victor_klemm/Documents/ÆFour Molecules/3D Molecules/47.png" ("path to PNG file") path "/Macintosh HD/Users/victor_klemm/Documents/ÆFour Molecules/3D Molecules/16.png" ("path to PNG file")] -> w414
          frame Default {
          }
          frame "1", "CH3CH3", "Ethan", "ethane" {
          }
          frame "2", "CH3CH2CH3", "Propan", "propane" {
          }
          frame "3", "Butan", "CH3(CH2)2CH3", "CH3CH2CH2CH3", "butane" {
          }
          frame "4", "CH3(CH2)3CH3", "CH3CH2CH2CH2CH3", "Pentan", "pentane" {
          }
          frame "5", "CH3CHCH2", "Propen", "propene" {
          }
          frame "6", "But-1-en", "CH3CH2CHCH2", "but-1-ene" {
          }
          frame "7", "CH3(CH2)2CHCH2", "CH3CH2CH2CHCH2", "Pent-1-en", "pent-1-ene" {
          }
          frame "8", "CH3NH2", "Methylamin", "methylamine" {
          }
          frame "9", "CH3CH2NH2", "Ethylamin", "ethylamine" {
          }
          frame "10", "CH3(CH2)2NH2", "CH3CH2CH2NH2", "Propyl-1-amin", "propyl-1-amine" {
          }
          frame "11", "Butyl-1-amin", "CH3(CH2)3NH2", "CH3CH2CH2CH2NH2", "butyl-1-amine" {
          }
          frame "12", "CH3OH", "Methanol", "methanol" {
          }
          frame "13", "CH3CH2OH", "Ethanol", "ethanol" {
          }
          frame "14", "CH3(CH2)2OH", "CH3CH2CH2OH", "Propanol", "propanol" {
          }
          frame "15", "Butanol", "CH3(CH2)3OH", "CH3CH2CH2CH2OH", "butanol" {
          }
          frame "16", "CH3CH2Cl", "Chlorethan", "chloroethane" {
          }
          frame "1-Chlorpropan", "1-chloropropane", "17", "CH3(CH2)2Cl", "CH3CH2CH2Cl" {
          }
          frame "1-Chlorbutan", "1-chlorobutane", "18", "CH3(CH2)3Cl", "CH3CH2CH2CH2Cl" {
          }
          frame "1-Chlorpentan", "1-chloropentane", "19", "CH3(CH2)4Cl", "CH3CH2CH2CH2CH2Cl" {
          }
          frame "20", "CH3CH2I", "Iodethan", "iodoethane" {
          }
          frame "1-Iodpropan", "1-iodopropane", "21", "CH3(CH2)2I", "CH3CH2CH2I" {
          }
          frame "1-Iodbutan", "1-iodobutane", "22", "CH3(CH2)3I", "CH3CH2CH2CH2I" {
          }
          frame "1-Iodpentan", "1-iodopentane", "23", "CH3(CH2)4I", "CH3CH2CH2CH2CH2I" {
          }
          frame "24", "Bromethan", "CH3CH2Br", "bromoethane" {
          }
          frame "1-Brompropan", "1-bromopropane", "25", "CH3(CH2)2Br", "CH3CH2CH2Br" {
          }
          frame "1-Brombutan", "1-bromobutane", "26", "CH3(CH2)3Br", "CH3CH2CH2CH2Br" {
          }
          frame "1-Brompentan", "1-bromopentane", "27", "CH3(CH2)4Br", "CH3CH2CH2CH2CH2Br" {
          }
          frame "28", "CH2CHNH2", "Ethenylamin", "ethenylamine" {
          }
          frame "29", "But-3-enyl-1-amin", "CH2CH(CH2)2NH2", "CH2CHCH2CH2NH2", "but-3-enyl-1-amine" {
          }
          frame "30", "CH2CHOH", "Ethenol", "ethenol" {
          }
          frame "31", "But-3-en-1-ol", "CH2CH(CH2)2OH", "CH2CHCH2CH2OH", "but-3-en-1-ol" {
          }
          frame "3-Chlorprop-1-en", "3-chloroprop-1-ene", "32", "CH2CHCH2Cl" {
          }
          frame "33", "5-Chlorpent-1-en", "5-chloropent-1-ene", "CH2CH(CH2)3Cl", "CH2CHCH2CH2CH2Cl" {
          }
          frame "3-Iodprop-1-en", "3-iodoprop-1-ene", "34", "CH2CHCH2I" {
          }
          frame "35", "5-Iodpent-1-en", "5-iodopent-1-ene", "CH2CH(CH2)3I", "CH2CHCH2CH2CH2I" {
          }
          frame "3-Bromprop-1-en", "3-bromoprop-1-ene", "36", "CH2CHCH2Br" {
          }
          frame "37", "5-Brompent-1-en", "5-bromopent-1-ene", "CH2CH(CH2)3Br", "CH2CHCH2CH2CH2Br" {
          }
          frame "38", "Aminomethanol", "NH2CH2OH", "aminomethanol" {
          }
          frame "3-Aminopropan-1-ol", "3-aminopropan-1-ol", "39", "NH2(CH2)3OH", "NH2CH2CH2CH2OH" {
          }
          frame "40", "Methandiol", "OHCH2OH", "methanediol" {
          }
          frame "41", "OH(CH2)3OH", "OHCH2CH2CH2OH", "Propan-1,3-diol", "propane-1,3-diol" {
          }
          frame "2-Chlorethan-1-ol", "2-chloroethan-1-ol", "42", "ClCH2CH2OH" {
          }
          frame "4-Chlorbutan-1-ol", "4-chlorbutan-1-ol", "43", "Cl(CH2)4OH", "ClCH2CH2CH2CH2OH" {
          }
          frame "2-Iodethan-1-ol", "2-iodoethan-1-ol", "44", "ICH2CH2OH" {
          }
          frame "4-Iodbutan-1-ol", "4-iodobutan-1-ol", "45", "I(CH2)4OH", "ICH2CH2CH2CH2OH" {
          }
          frame "2-Bromethan-1-ol", "2-bromoethan-1-ol", "46", "BrCH2CH2OH" {
          }
          frame "4-Brombutan-1-ol", "4-bromobutan-1-ol", "47", "Br(CH2)4OH", "BrCH2CH2CH2CH2OH" {
          }
          frame "T" {
          }
        }
        n95 = local read "Status:"() -> (w413:string)
        n96 = call <vilib>:"Read PNG File.vi"("path to PNG file"=w414) -> ("image data"=w418:T3)  [unwired: 8 in, 2 out]
        n97 = call <vilib>:"Read PNG File.vi"("path to PNG file"=w415) -> ("image data"=w416:T3)  [unwired: 8 in, 2 out]
        n98 = Array Size(array=w420) -> (size(s)=w422:i32)
        n99 = Index Array(array=w420, index=w423) -> (element=w393:dbl)
        n100 = call <vilib>:"Draw Flattened Pixmap.vi"("image data"=w418) -> ("new picture"=→"3D-Image":picture)  [unwired: 8 in]
        n101 = call <vilib>:"Draw Flattened Pixmap.vi"("image data"=w416) -> ("new picture"=→"2D-Image":picture)  [unwired: 8 in]
        n102 = case shown="22" w393 {
          tunnel: [FALSE TRUE FALSE FALSE FALSE FALSE FALSE FALSE FALSE FALSE FALSE FALSE FALSE FALSE FALSE FALSE FALSE FALSE FALSE FALSE FALSE FALSE FALSE FALSE] -> w426
          tunnel: [dbl[] [] ("array") dbl[] [] ("array") dbl[] [360.0, 730.0, 360.0, 685.0, 0.0] ("array") dbl[] [420.0, 570.0, 320.0, 690.0, 0.0] ("array") dbl[] [485.0, 470.0, 320.0, 680.0, 0.0] ("array") dbl[] [585.0, 395.0, 325.0, 690.0, 0.0] ("array") dbl[] [770.0, 375.0, 375.0, 705.0, 0.0] ("array") dbl[] [365.0, 740.0, 680.0, 350.0, 0.0] ("array") dbl[] [420.0, 580.0, 680.0, 325.0, 0.0] ("array") dbl[] [485.0, 470.0, 680.0, 320.0, 0.0] ("array") dbl[] [585.0, 395.0, 690.0, 340.0, 0.0] ("array") dbl[] [735.0, 365.0, 700.0, 395.0, 0.0] ("array") dbl[] [315.0, 705.0, 465.0, 465.0, 0.0] ("array") dbl[] [345.0, 580.0, 427.0, 427.0, 0.0] ("array") dbl[] [610.0, 345.0, 452.0, 452.0, 0.0] ("array") dbl[] [720.0, 315.0, 505.0, 505.0, 0.0] ("array") dbl[] [480.0, 475.0, 380.0, 500.0, 0.0] ("array") dbl[] [425.0, 425.0, 390.0, 460.0, 0.0] ("array") dbl[] [463.0, 458.0, 458.0, 465.0, 0.0] ("array") dbl[] [395.0, 395.0, 430.0, 385.0, 0.0] ("array") dbl[] [500.0, 500.0, 490.0, 400.0, 0.0] ("array") dbl[] [495.0, 475.0, 380.0, 500.0, 0.0] ("array") dbl[] [435.0, 435.0, 445.0, 385.0, 0.0] ("array") dbl[] [410.0, 410.0, 390.0, 460.0, 0.0] ("array")] -> w421
          tunnel: [FALSE FALSE TRUE TRUE TRUE TRUE TRUE TRUE TRUE TRUE TRUE TRUE TRUE TRUE TRUE TRUE FALSE FALSE FALSE FALSE FALSE FALSE FALSE FALSE] -> w424
          frame Default {
          }
          frame 0 {
            n103 = local write "Status:"("Finished!" ("Status:")) -> ()
          }
          frame 1 {
          }
          frame 2 {
          }
          frame 3 {
          }
          frame 4 {
          }
          frame 5 {
          }
          frame 6 {
          }
          frame 7 {
          }
          frame 8 {
          }
          frame 9 {
          }
          frame 10 {
          }
          frame 11 {
          }
          frame 12 {
          }
          frame 13 {
          }
          frame 14 {
          }
          frame 15 {
          }
          frame 16 {
          }
          frame 17 {
          }
          frame 18 {
          }
          frame 19 {
          }
          frame 20 {
          }
          frame 21 {
          }
          frame 22 {
          }
        }
        n104 = case shown="\"Building...\"" w413 {
          tunnel: [w437 w457 w497 w498] -> w412
          tunnel: [w437 w451 w497 w498] -> w411
          tunnel: [w437 w448 w497 w498] -> w410
          tunnel: [w437 w439 w497 w498] -> w409
          tunnel: [w437 w453 w497 w498] -> w408
          tunnel: [w437 w449 w497 w498] -> w407
          tunnel: [w437 w445 w497 w498] -> w406
          tunnel: [w437 w442 w497 w498] -> w405
          tunnel: [w437 w456 w497 w498] -> w404
          tunnel: [w437 w452 w497 w498] -> w403
          tunnel: [w437 w446 w497 w498] -> w402
          tunnel: [w437 w444 w497 w498] -> w401
          tunnel: [w437 w455 w497 w498] -> w394
          tunnel: [w437 w447 w497 w498] -> w400
          tunnel: [w437 w450 w497 w498] -> w399
          tunnel: [w437 w443 w497 w498] -> w398
          tunnel: [w437 w440 w497 w498] -> w397
          tunnel: [w437 w454 w497 w498] -> w396
          tunnel: [w437 w441 w497 w498] -> w395
          tunnel: w393 -> [_ w438 _ _]
          frame Default {
            w437 = FALSE
          }
          frame "Building..." {
            n105 = case shown="19" w438 {
              tunnel: [w458 TRUE ("stop? (T)") w461 w463 w465 w467 w469 w471 w473 w475 w477 w479 w481 w483 w485 w487 w489 w491 w494 w495] -> w457
              tunnel: [w458 w459 w461 w463 w465 w467 w469 w471 w473 w475 TRUE ("stop? (T)") w479 w481 w483 w485 w487 w489 w491 w494 w495] -> w456
              tunnel: [w458 w459 w461 w463 w465 w467 w469 w471 w473 w475 w477 w479 w481 w483 TRUE ("stop? (T)") w487 w489 w491 w494 w495] -> w455
              tunnel: [w458 w459 w461 w463 w465 w467 w469 w471 w473 w475 w477 w479 w481 w483 w485 w487 w489 w491 w494 TRUE ("stop? (T)")] -> w454
              tunnel: [w458 w459 w461 w463 w465 w467 TRUE ("stop? (T)") w471 w473 w475 w477 w479 w481 w483 w485 w487 w489 w491 w494 w495] -> w453
              tunnel: [w458 w459 w461 w463 w465 w467 w469 w471 w473 w475 w477 TRUE ("stop? (T)") w481 w483 w485 w487 w489 w491 w494 w495] -> w452
              tunnel: [w458 w459 TRUE ("stop? (T)") w463 w465 w467 w469 w471 w473 w475 w477 w479 w481 w483 w485 w487 w489 w491 w494 w495] -> w451
              tunnel: [w458 w459 w461 w463 w465 w467 w469 w471 w473 w475 w477 w479 w481 w483 w485 w487 TRUE ("stop? (T)") w491 w494 w495] -> w450
              tunnel: [w458 w459 w461 w463 w465 w467 w469 TRUE ("stop? (T)") w473 w475 w477 w479 w481 w483 w485 w487 w489 w491 w494 w495] -> w449
              tunnel: [w458 w459 w461 TRUE ("stop? (T)") w465 w467 w469 w471 w473 w475 w477 w479 w481 w483 w485 w487 w489 w491 w494 w495] -> w448
              tunnel: [w458 w459 w461 w463 w465 w467 w469 w471 w473 w475 w477 w479 w481 w483 w485 TRUE ("stop? (T)") w489 w491 w494 w495] -> w447
              tunnel: [w458 w459 w461 w463 w465 w467 w469 w471 w473 w475 w477 w479 TRUE ("stop? (T)") w483 w485 w487 w489 w491 w494 w495] -> w446
              tunnel: [w458 w459 w461 w463 w465 w467 w469 w471 TRUE ("stop? (T)") w475 w477 w479 w481 w483 w485 w487 w489 w491 w494 w495] -> w445
              tunnel: [w458 w459 w461 w463 w465 w467 w469 w471 w473 w475 w477 w479 w481 TRUE ("stop? (T)") w485 w487 w489 w491 w494 w495] -> w444
              tunnel: [w458 w459 w461 w463 w465 w467 w469 w471 w473 w475 w477 w479 w481 w483 w485 w487 w489 TRUE ("stop? (T)") w494 w495] -> w443
              tunnel: [w458 w459 w461 w463 w465 w467 w469 w471 w473 TRUE ("stop? (T)") w477 w479 w481 w483 w485 w487 w489 w491 w494 w495] -> w442
              tunnel: [w458 w459 w461 w463 TRUE ("stop? (T)") w467 w469 w471 w473 w475 w477 w479 w481 w483 w485 w487 w489 w491 w494 w495] -> w441
              tunnel: [w458 w459 w461 w463 w465 w467 w469 w471 w473 w475 w477 w479 w481 w483 w485 w487 w489 w491 TRUE ("stop? (T)") w495] -> w440
              tunnel: [w458 w459 w461 w463 w465 TRUE ("stop? (T)") w469 w471 w473 w475 w477 w479 w481 w483 w485 w487 w489 w491 w494 w495] -> w439
              frame 0, Default {
                w458 = FALSE ("stop? (T)")
              }
              frame 1 {
                w459 = FALSE ("stop? (T)")
              }
              frame 2 {
                w461 = FALSE ("stop? (T)")
              }
              frame 3 {
                w463 = FALSE ("stop? (T)")
              }
              frame 4 {
                w465 = FALSE ("stop? (T)")
              }
              frame 5 {
                w467 = FALSE ("stop? (T)")
              }
              frame 6 {
                w469 = FALSE ("stop? (T)")
              }
              frame 7 {
                w471 = FALSE ("stop? (T)")
              }
              frame 8 {
                w473 = FALSE ("stop? (T)")
              }
              frame 9 {
                w475 = FALSE ("stop? (T)")
              }
              frame 10 {
                w477 = FALSE ("stop? (T)")
              }
              frame 11 {
                w479 = FALSE ("stop? (T)")
              }
              frame 12 {
                w481 = FALSE ("stop? (T)")
              }
              frame 13 {
                w483 = FALSE ("stop? (T)")
              }
              frame 14 {
                w485 = FALSE ("stop? (T)")
              }
              frame 15, 20 {
                w487 = FALSE ("stop? (T)")
              }
              frame 16, 22 {
                w489 = FALSE ("stop? (T)")
              }
              frame 17 {
                w491 = FALSE ("stop? (T)")
              }
              frame 18, 21 {
                w494 = FALSE ("stop? (T)")
              }
              frame 19 {
                w495 = FALSE ("stop? (T)")
              }
            }
          }
          frame "Finished!" {
            w497 = FALSE
          }
          frame "Stop" {
            w498 = FALSE ("stop? (T)")
          }
        }
        "?" <- w399
        "?" <- w398
        "?" <- w397
        "?" <- w396
        "?" <- w401
        "?" <- w394
        "?" <- w400
        "?" <- w402
        "?" <- w403
        "?" <- w404
        "?" <- w405
        "?" <- w406
        "?" <- w407
        "?" <- w408
        "?" <- w409
        "?" <- w395
        "?" <- w410
        "?" <- w411
        "?" <- w412
        n106 = Index Array(array=w421, index #1=0 ("index"), index #2=1 ("index"), index #3=2 ("index"), index #4=3 ("index")) -> (element #1=w431:dbl, element #2=w430:dbl, element #3=w429:dbl, element #4=w432:dbl)
      }
    }
    n107 = Negate(x=w270) -> (-x=w269:dbl)
    n108 = Negate(x=w268) -> (-x=w267:dbl)
    n109 = Negate(x=w266) -> (-x=w265:dbl)
    n110 = Negate(x=w264) -> (-x=w263:dbl)
    n111 = Add(x=w273, y=1) -> (x+y=w271:i32)
    n112 = Divide(x=100.0 ("y"), y=w274) -> (x/y=w277:dbl)
    n113 = Multiply(x=w277, y=w271) -> (x*y=w276:dbl)
    n114 = case shown="False" w279 {
      tunnel: w263 -> [w297 _]
      tunnel: w269 -> [w300 _]
      tunnel: w267 -> [w299 _]
      tunnel: w265 -> [w298 _]
      tunnel: w287 -> [w291 w392]
      tunnel: w286 -> [w290 w391]
      tunnel: w280 -> [w292 _]
      tunnel: [w294 w392] -> w262
      tunnel: [w293 w391] -> w261
      frame False {
        # "Der Greifer šffnet sich"
        # "Die Motoren drehen, bis sie den gewŸnschten Winkel erreichen"
        # "Der Greifer šffnet oder schliesst sich"
        # "Die Motoren werden wieder in die Grundposition verschoben"
        n115 = case shown="True" w292 {
          tunnel: w291 -> [w304 w308]
          tunnel: w290 -> [w303 w307]
          tunnel: [w304 w306] -> w289
          tunnel: [w303 w305] -> w288
          frame False {
          }
          frame True {
            n116 = flat-sequence {
              tunnel: [w309] -> w306
              tunnel: [w312] -> w305
              tunnel: w308 -> [w314]
              tunnel: w307 -> [w312]
              frame #0 {
                w316 = T4 2 items=["Port A"=0, "Port B"=1, "Port C"=2, "Ports A & B"=4, "Ports A & C"=5, "Ports B & C"=6, "All Ports"=3] ("Output Port (All Ports)")
                n117 = call <vilib>:"Wait_Num.vi"("Time (1 sec)"=sgl 1.0, "NXT"=w314) -> ("NXT"=w313:T2)  [unwired: 2 in]
                n118 = call <vilib>:"MotorOn.vi"("Power (75)"=50, "NXT"=w313, "Output Port (All Ports)"=w316) -> ("NXT"=w310:T2)  [unwired: 1 in]
                n119 = call <vilib>:"Wait_Num.vi"("Time (1 sec)"=sgl 1.0, "NXT"=w310) -> ("NXT"=w309:T2)  [unwired: 2 in]
              }
            }
          }
        }
        n120 = flat-sequence {
          tunnel: w288 -> [w364]
          tunnel: w289 -> [w344]
          tunnel: [w351] -> w301
          tunnel: [w350] -> w302
          tunnel: w300 -> [w348]
          tunnel: w299 -> [w347]
          tunnel: w298 -> [w346]
          tunnel: w297 -> [w345]
          frame #0 {
            w349 = -30 ("Power (75)")
            w355 = T4 1 items=["Port A"=0, "Port B"=1, "Port C"=2, "Ports A & B"=4, "Ports A & C"=5, "Ports B & C"=6, "All Ports"=3] ("Output Port (All Ports)")
            w354 = T4 0 items=["Port A"=0, "Port B"=1, "Port C"=2, "Ports A & B"=4, "Ports A & C"=5, "Ports B & C"=6, "All Ports"=3] ("Output Port (All Ports)")
            w352 = T4 1 items=["Port A"=0, "Port B"=1, "Port C"=2, "Ports A & B"=4, "Ports A & C"=5, "Ports B & C"=6, "All Ports"=3] ("Output Port (All Ports)")
            w356 = T4 0 items=["Port A"=0, "Port B"=1, "Port C"=2, "Ports A & B"=4, "Ports A & C"=5, "Ports B & C"=6, "All Ports"=3] ("Output Port (All Ports)")
            n121 = call <vilib>:"MotorOn.vi"("Power (75)"=w349, "NXT"=w364, "Output Port (All Ports)"=w356) -> ("NXT"=w363:T2)  [unwired: 1 in]
            n122 = call <vilib>:"MotorOn.vi"("Power (75)"=w349, "NXT"=w364, "Output Port (All Ports)"=w352) -> ("NXT"=w360:T2)  [unwired: 1 in]
            n123 = call <vilib>:"MotorOn.vi"("Power (75)"=w349, "NXT"=w344, "Output Port (All Ports)"=w354) -> ("NXT"=w361:T2)  [unwired: 1 in]
            n124 = call <vilib>:"MotorOn.vi"("Power (75)"=w349, "NXT"=w344, "Output Port (All Ports)"=w355) -> ("NXT"=w362:T2)  [unwired: 1 in]
            n125 = call <vilib>:"Wait_Rotation.vi"("Position Change (180)"=w346, "NXT"=w363, "Port (Port A)"=w356) -> ("NXT"=w357:T2)  [unwired: 1 in]
            n126 = call <vilib>:"Wait_Rotation.vi"("Position Change (180)"=w345, "NXT"=w360, "Port (Port A)"=w352) -> ("NXT"=w353:T2)  [unwired: 1 in]
            n127 = call <vilib>:"Wait_Rotation.vi"("Position Change (180)"=w348, "NXT"=w361, "Port (Port A)"=w354) -> ("NXT"=w359:T2)  [unwired: 1 in]
            n128 = call <vilib>:"Wait_Rotation.vi"("Position Change (180)"=w347, "NXT"=w362, "Port (Port A)"=w355) -> ("NXT"=w358:T2)  [unwired: 1 in]
            n129 = call <vilib>:"MotorBrake.vi"("NXT"=w357, "Port (All Ports)"=w356) -> ()  [unwired: 2 in, 1 out]
            n130 = call <vilib>:"MotorBrake.vi"("NXT"=w353, "Port (All Ports)"=w352) -> ("NXT"=w351:T2)  [unwired: 2 in]
            n131 = call <vilib>:"MotorBrake.vi"("NXT"=w359, "Port (All Ports)"=w354) -> ()  [unwired: 2 in, 1 out]
            n132 = call <vilib>:"MotorBrake.vi"("NXT"=w358, "Port (All Ports)"=w355) -> ("NXT"=w350:T2)  [unwired: 2 in]
          }
        }
        n133 = case shown="False" w292 {
          tunnel: w302 -> [w321 w334]
          tunnel: w301 -> [w320 w333]
          tunnel: [w319 w332] -> w296
          tunnel: [w318 w331] -> w295
          frame False {
            n134 = flat-sequence {
              tunnel: [w322] -> w319
              tunnel: [w325] -> w318
              tunnel: w321 -> [w327]
              tunnel: w320 -> [w325]
              frame #0 {
                w329 = T4 2 items=["Port A"=0, "Port B"=1, "Port C"=2, "Ports A & B"=4, "Ports A & C"=5, "Ports B & C"=6, "All Ports"=3] ("Output Port (All Ports)")
                n135 = call <vilib>:"Wait_Num.vi"("Time (1 sec)"=sgl 1.0, "NXT"=w327) -> ("NXT"=w326:T2)  [unwired: 2 in]
                n136 = call <vilib>:"MotorOn.vi"("Power (75)"=9, "NXT"=w326, "Output Port (All Ports)"=w329) -> ("NXT"=w323:T2)  [unwired: 1 in]
                n137 = call <vilib>:"Wait_Num.vi"("Time (1 sec)"=sgl 1.0, "NXT"=w323) -> ("NXT"=w322:T2)  [unwired: 2 in]
              }
            }
          }
          frame True {
            n138 = flat-sequence {
              tunnel: w333 -> [w337]
              tunnel: [w336] -> w332
              tunnel: w334 -> [w340]
              tunnel: [w337] -> w331
              frame #0 {
                w341 = T4 2 items=["Port A"=0, "Port B"=1, "Port C"=2, "Ports A & B"=4, "Ports A & C"=5, "Ports B & C"=6, "All Ports"=3] ("Output Port (All Ports)")
                n139 = call <vilib>:"Wait_Num.vi"("Time (1 sec)"=sgl 1.0, "NXT"=w340) -> ("NXT"=w339:T2)  [unwired: 2 in]
                n140 = call <vilib>:"MotorOn.vi"("Power (75)"=-100, "NXT"=w339, "Output Port (All Ports)"=w341) -> ("NXT"=w335:T2)  [unwired: 1 in]
                n141 = call <vilib>:"Wait_Num.vi"("Time (1 sec)"=sgl 1.0, "NXT"=w335) -> ("NXT"=w336:T2)  [unwired: 2 in]
              }
            }
          }
        }
        n142 = flat-sequence {
          tunnel: w296 -> [w386]
          tunnel: w295 -> [w385]
          tunnel: [w372] -> w294
          tunnel: [w371] -> w293
          frame #0 {
            w365 = u16 500 ("Tone (440 Hz)")
            w368 = T4 1 items=["Port A"=0, "Port B"=1, "Port C"=2, "Ports A & B"=4, "Ports A & C"=5, "Ports B & C"=6, "All Ports"=3] ("Output Port (All Ports)")
            w381 = T5 1 items=["Port 1", "Port 2", "Port 3", "Port 4"] ("Port (Port 1)")
            w380 = T5 0 items=["Port 1", "Port 2", "Port 3", "Port 4"] ("Port (Port 1)")
            w366 = T4 1 items=["Port A"=0, "Port B"=1, "Port C"=2, "Ports A & B"=4, "Ports A & C"=5, "Ports B & C"=6, "All Ports"=3] ("Output Port (All Ports)")
            w367 = T4 0 items=["Port A"=0, "Port B"=1, "Port C"=2, "Ports A & B"=4, "Ports A & C"=5, "Ports B & C"=6, "All Ports"=3] ("Output Port (All Ports)")
            w369 = T5 1 items=["Port 1", "Port 2", "Port 3", "Port 4"] ("Port (Port 1)")
            w382 = T5 0 items=["Port 1", "Port 2", "Port 3", "Port 4"] ("Port (Port 1)")
            w373 = 30 ("Power (75)")
            w370 = T4 0 items=["Port A"=0, "Port B"=1, "Port C"=2, "Ports A & B"=4, "Ports A & C"=5, "Ports B & C"=6, "All Ports"=3] ("Output Port (All Ports)")
            n143 = call <vilib>:"MotorOn.vi"("Power (75)"=w373, "NXT"=w385, "Output Port (All Ports)"=w366) -> ("NXT"=w387:T2)  [unwired: 1 in]
            n144 = call <vilib>:"MotorOn.vi"("Power (75)"=w373, "NXT"=w385, "Output Port (All Ports)"=w367) -> ("NXT"=w388:T2)  [unwired: 1 in]
            n145 = call <vilib>:"MotorOn.vi"("Power (75)"=w373, "NXT"=w386, "Output Port (All Ports)"=w370) -> ("NXT"=w390:T2)  [unwired: 1 in]
            n146 = call <vilib>:"MotorOn.vi"("Power (75)"=w373, "NXT"=w386, "Output Port (All Ports)"=w368) -> ("NXT"=w389:T2)  [unwired: 1 in]
            n147 = call <vilib>:"Wait_Touch.vi"("NXT"=w387, "Port (Port 1)"=w381) -> ("NXT"=w377:T2)  [unwired: 2 in]
            n148 = call <vilib>:"Wait_Touch.vi"("NXT"=w388, "Port (Port 1)"=w380) -> ("NXT"=w375:T2)  [unwired: 2 in]
            n149 = call <vilib>:"Wait_Touch.vi"("NXT"=w390, "Port (Port 1)"=w382) -> ("NXT"=w384:T2)  [unwired: 2 in]
            n150 = call <vilib>:"Wait_Touch.vi"("NXT"=w389, "Port (Port 1)"=w369) -> ("NXT"=w379:T2)  [unwired: 2 in]
            n151 = call <vilib>:"Tone.vi"("NXT"=w377) -> ("NXT"=w376:T2)  [unwired: 3 in]
            n152 = call <vilib>:"Tone.vi"("NXT"=w375, "Tone (440 Hz)"=w365) -> ("NXT"=w374:T2)  [unwired: 2 in]
            n153 = call <vilib>:"Tone.vi"("NXT"=w384) -> ("NXT"=w383:T2)  [unwired: 3 in]
            n154 = call <vilib>:"Tone.vi"("NXT"=w379, "Tone (440 Hz)"=w365) -> ("NXT"=w378:T2)  [unwired: 2 in]
            n155 = call <vilib>:"MotorBrake.vi"("NXT"=w376, "Port (All Ports)"=w366) -> ()  [unwired: 2 in, 1 out]
            n156 = call <vilib>:"MotorBrake.vi"("NXT"=w374, "Port (All Ports)"=w367) -> ("NXT"=w371:T2)  [unwired: 2 in]
            n157 = call <vilib>:"MotorBrake.vi"("NXT"=w383, "Port (All Ports)"=w370) -> ("NXT"=w372:T2)  [unwired: 2 in]
            n158 = call <vilib>:"MotorBrake.vi"("NXT"=w378, "Port (All Ports)"=w368) -> ()  [unwired: 2 in, 1 out]
          }
        }
      }
      frame True {
      }
    }
    n159 = Round To Nearest(number=w276) -> (nearest integer value=→"Progress":dbl)
  }
  n160 = flat-sequence {
    tunnel: w4 -> [w735]
    tunnel: [w733] -> w3
    tunnel: w5 -> [w731]
    tunnel: [w730] -> w6
    frame #0 {
      w732 = T4 4 items=["Port A"=0, "Port B"=1, "Port C"=2, "Ports A & B"=4, "Ports A & C"=5, "Ports B & C"=6, "All Ports"=3] ("Output Port (All Ports)")
      w734 = T4 4 items=["Port A"=0, "Port B"=1, "Port C"=2, "Ports A & B"=4, "Ports A & C"=5, "Ports B & C"=6, "All Ports"=3] ("Output Port (All Ports)")
      n161 = call <vilib>:"MotorCoast.vi"("NXT"=w731, "Port (All Ports)"=w732) -> ("NXT"=w730:T2)  [unwired: 2 in]
      n162 = call <vilib>:"MotorCoast.vi"("NXT"=w735, "Port (All Ports)"=w734) -> ("NXT"=w733:T2)  [unwired: 2 in]
    }
  }
  n163 = flat-sequence {
    tunnel: w3 -> [w739]
    tunnel: [w737] -> w18
    tunnel: w6 -> [w736]
    tunnel: [w736] -> w9
    frame #0 {
      w738 = T4 2 items=["Port A"=0, "Port B"=1, "Port C"=2, "Ports A & B"=4, "Ports A & C"=5, "Ports B & C"=6, "All Ports"=3] ("Output Port (All Ports)")
      n164 = call <vilib>:"MotorCoast.vi"("NXT"=w739, "Port (All Ports)"=w738) -> ("NXT"=w737:T2)  [unwired: 2 in]
    }
  }
  n165 = flat-sequence {
    tunnel: w18 -> [w743]
    tunnel: [w740] -> w2
    tunnel: [w742] -> w1
    tunnel: w9 -> [w741]
    frame #0 {
      n166 = while {
        tunnel: w743 -> [w747]
        tunnel: w741 -> [w746]
        tunnel: [w747] -> w742
        tunnel: [w745] -> w740
        i -> [w748]
        stop <- "?" stop-if-true
        n167 = Divide(x=w748, y=2) -> (x/y=w751:dbl)
        n168 = Wait (ms)(milliseconds to wait=u32 500) -> ()  [unwired: 1 out]
        n169 = Round To Nearest(number=w751) -> (nearest integer value=w750:dbl)
        n170 = Equal?(x=w750, y=w751) -> (x = y?=w752:bool)
        n171 = case shown="True" w752 {
          tunnel: w746 -> [w755 w759]
          tunnel: [w754 w757] -> w745
          frame False {
            w756 = T4 2 items=["Port A"=0, "Port B"=1, "Port C"=2, "Ports A & B"=4, "Ports A & C"=5, "Ports B & C"=6, "All Ports"=3] ("Port (All Ports)")
            n172 = call <vilib>:"MotorCoast.vi"("NXT"=w755, "Port (All Ports)"=w756) -> ("NXT"=w754:T2)  [unwired: 2 in]
          }
          frame True {
            w758 = T4 2 items=["Port A"=0, "Port B"=1, "Port C"=2, "Ports A & B"=4, "Ports A & C"=5, "Ports B & C"=6, "All Ports"=3] ("Output Port (All Ports)")
            n173 = call <vilib>:"MotorOn.vi"("Power (75)"=100, "NXT"=w759, "Output Port (All Ports)"=w758) -> ("NXT"=w757:T2)  [unwired: 1 in]
          }
        }
      }
    }
  }
  n174 = flat-sequence {
    tunnel: [w765] -> w14
    tunnel: w1 -> [w765]
    tunnel: [w761] -> w16
    tunnel: w2 -> [w762]
    frame #0 {
      w763 = T4 2 items=["Port A"=0, "Port B"=1, "Port C"=2, "Ports A & B"=4, "Ports A & C"=5, "Ports B & C"=6, "All Ports"=3] ("Port (All Ports)")
      n175 = local write "Status:"("Stop" ("Status:")) -> ()
      n176 = Wait (ms)(milliseconds to wait=u32 1000) -> ()  [unwired: 1 out]
      n177 = call <vilib>:"MotorCoast.vi"("NXT"=w762, "Port (All Ports)"=w763) -> ("NXT"=w761:T2)  [unwired: 2 in]
    }
  }
  n178 = flat-sequence {
    tunnel: [w774] -> w17
    tunnel: w16 -> [w774]
    tunnel: [w773] -> w15
    tunnel: w14 -> [w773]
    frame #0 {
      w771 = "" ("Status:")
      n179 = local write "Progress"(u8 0 ("Progress")) -> ()
      n180 = local write "2D-Image"(picture data[5B] ("2D")) -> ()
      n181 = local write "Status:"(w771) -> ()
      n182 = local write "Input molecule name or extended sum formula:"(w771) -> ()
      n183 = call <vilib>:"Read PNG File.vi"("path to PNG file"=path "/Macintosh HD/Users/victor_klemm/Documents/ÆFour Molecules/3D Molecules/0.png") -> ("image data"=w770:T3)  [unwired: 8 in, 2 out]
      n184 = call <vilib>:"Draw Flattened Pixmap.vi"("image data"=w770) -> ("new picture"=w768:picture)  [unwired: 8 in]
      n185 = local write "3D-Image"(w768) -> ()
    }
  }
  n186 = flat-sequence {
    tunnel: w17 -> [_]
    tunnel: w15 -> [_]
    frame #0 {
      n187 = Stop(stop? (T)=TRUE) -> ()
    }
  }
